vi "poly_xwav2xy_single.vi"(7 "XY graph":refnum<vi>, 8 "error in":errorcluster, 9 "plot index (0)":i32, 10 "relative x? (F)":bool, 11 "xwave":T1={"attributes"=variant, "X"={"start"=0.0, "delta"=0.0, "units"="index", "dim"="au"}, "Y"={"data"=[], "units"="au"}}) -> (0 "error out":errorcluster, 1 "xy cluster":cluster{"X":dbl[], "Y":dbl[]}, 2 "y units":string, 3 "x units":string, 4 "x dimention":string)   [LabVIEW 2015, in "_xwav_polys.lvlib"]
uses:
  _xwav_polys.lvlib
  xwav.ctl
  <vilib>/Utility/Data Type/NI_Data Type.lvlib
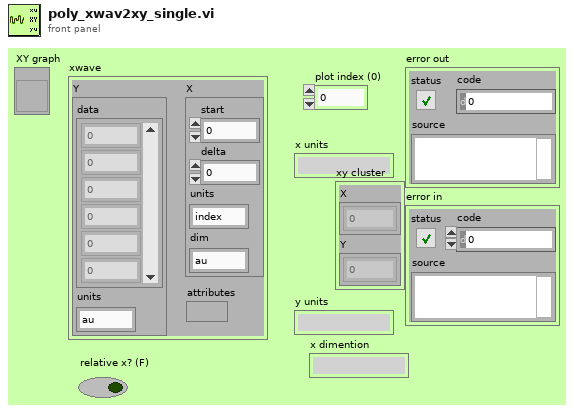
[diagram p1: front panel]
types:
  T1 = typedef "xwav.ctl" = cluster{"attributes":variant, "X":cluster{"start":dbl, "delta":dbl, "units":string, "dim":string}, "Y":cluster{"data":dbl[], "units":string}}
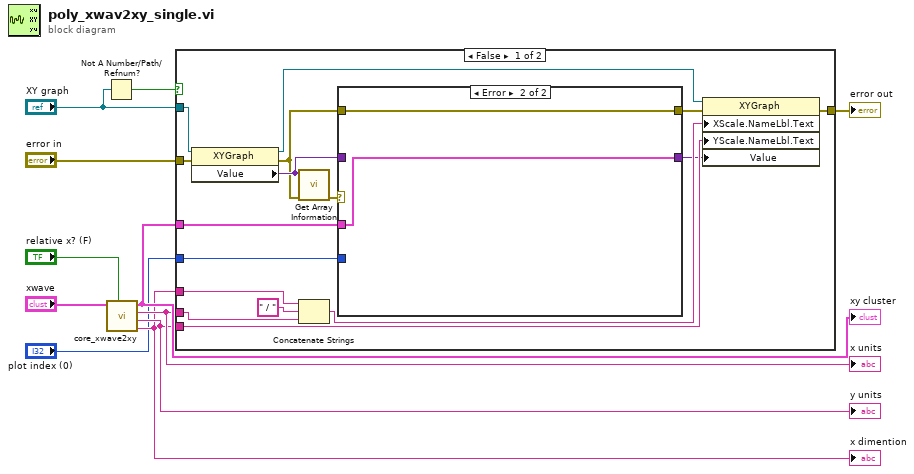
[diagram p0: block diagram]
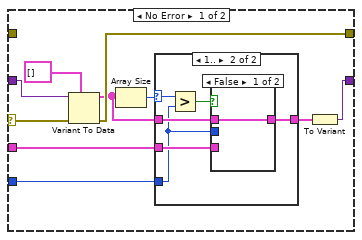
[diagram p2: hidden frame]
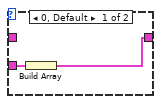
[diagram p3: hidden frame]
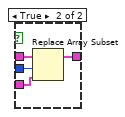
[diagram p4: hidden frame]
diagram:
  n1 = Not A Number/Path/Refnum?(number/path/refnum="XY graph") -> (NaN/Path/Refnum?=w11:bool)
  n2 = call "core_xwave2xy.vi"("relative x? (F)"="relative x? (F)", "xwave"="xwave") -> ("x dimention"=w2:string, "y units"=w3:string, "x units"=w4:string, "xy cluster"=w5:cluster{"X":dbl[], "Y":dbl[]})  [unwired: 6 in]
  "x units" <- w4
  "y units" <- w3
  "xy cluster" <- w5
  "x dimention" <- w2
  n3 = case shown="False" w11 {
    tunnel: "XY graph" -> [w21 _]
    tunnel: w5 -> [w16 _]
    tunnel: w4 -> [w26 _]
    tunnel: w2 -> [w25 _]
    tunnel: [w23 w53] -> w9
    tunnel: "error in" -> [w20 w53]
    tunnel: w3 -> [w22 _]
    tunnel: "plot index (0)" -> [w15 _]
    frame False {
      n4 = property class="XYGraph"(reference=w21, error in=w20) -> (reference out=w19:refnum<vi>, error out=w12:errorcluster, "Value"=w17:variant)
      n5 = call <vilib>:"Get Array Information.vi"("error in (no error)"=w12, "Variant"=w17) -> ("error out"=w18:errorcluster)  [unwired: 6 in, 3 out]
      n6 = Concatenate Strings(w25, " / " ("string"), w26) -> (w24:string)
      n7 = case shown="Error" w18 {
        selector: w18 -> [w31 _]
        tunnel: w17 -> [w36 _]
        tunnel: w16 -> [w34 w51]
        tunnel: w15 -> [w35 _]
        tunnel: [w32 w51] -> w14
        tunnel: [w30 w52] -> w13
        tunnel: w12 -> [_ w52]
        frame No Error {
          n8 = Variant To Data(error in=w31, type=cluster{dbl[], dbl[]}[] [] ("appended array"), Variant=w36) -> (data=w29:cluster{dbl[], dbl[]}[], error out=w30:errorcluster)
          n9 = Array Size(array=w29) -> (size(s)=w28:i32)
          n10 = case shown="1.." w28 {
            selector: w28 -> [_ w42]
            tunnel: w35 -> [_ w41]
            tunnel: w34 -> [w39 w45]
            tunnel: [w38 w44] -> w33
            tunnel: w29 -> [_ w43]
            frame 0, Default {
              n11 = Build Array(w39) -> (w38:cluster{"X":dbl[], "Y":dbl[]}[])
            }
            frame 1.. {
              n12 = Greater?(x=w42, y=w41) -> (0:w40:bool)
              n13 = case shown="False" w40 {
                tunnel: w41 -> [_ w50]
                tunnel: w45 -> [_ w49]
                tunnel: [w46 w48] -> w44
                tunnel: w43 -> [w46 w47]
                frame False {
                }
                frame True {
                  n14 = Replace Array Subset(array=w47, new element=w49, index=w50) -> (w48:cluster{dbl[], dbl[]}[])
                }
              }
            }
          }
          n15 = To Variant(anything=w33) -> (Variant=w32:variant)
        }
        frame Error {
        }
      }
      n16 = property class="XYGraph"(reference=w19, error in=w13, "XScale.NameLbl.Text"=w24, "YScale.NameLbl.Text"=w22, "Value"=w14) -> (error out=w23:errorcluster)  [unwired: 1 out]
    }
    frame True {
    }
  }
  "error out" <- w9
